vi "Read TopRef.vi"(8 "error in (no error)":errorcluster, 11 "UIActorTop2 in":refnum<class "UI_Top_Customer.lvclass">) -> (0 "error out":errorcluster, 2 "TopRef":T1, 3 "UIActorTop2 out":refnum<class "UI_Top_Customer.lvclass">)   [LabVIEW 2021, in "UI_Top_Customer.lvclass"]
uses:
  UI_Top_Customer.lvclass
  TopRef.ctl
  Buttons.ctl
  Launcher/Min Button.ctl
  UI_Top_Customer.lvclass/UI_Top_Customer.ctl
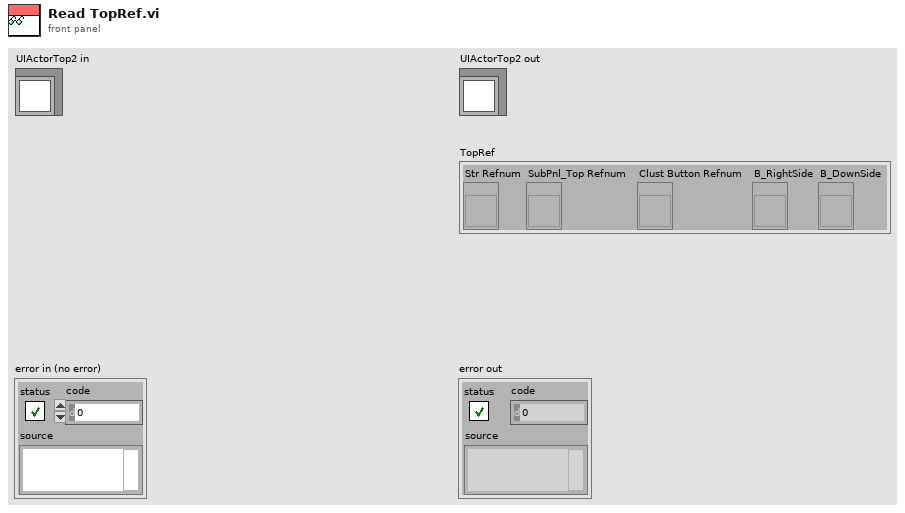
[diagram p1: front panel]
types:
  T1 = typedef "UI_Top_Customer.lvclass/TopRef.ctl" = cluster{"Str Refnum":refnum<vi>, "SubPnl_Top Refnum":refnum<vi>, "Clust Button Refnum":refnum<vi>, "B_RightSide":refnum<vi>, "B_DownSide":refnum<vi>}
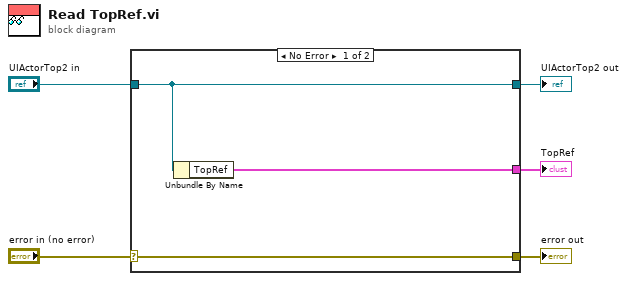
[diagram p0: block diagram]
diagram:
  n1 = case shown="No Error" "error in (no error)" {
    selector: "error in (no error)" -> [w8 w9]
    tunnel: [w8 w9] -> w4
    tunnel: [w7 w10] -> w2
    tunnel: "UIActorTop2 in" -> [w7 w10]
    tunnel: [w6 _] -> w1
    frame No Error {
      n2 = Unbundle By Name(w7) -> ("TopRef"=w6:T1)
    }
    frame Error {
    }
  }
  "error out" <- w4
  "UIActorTop2 out" <- w2
  "TopRef" <- w1
